vi "logo.vi"() -> ()   [LabVIEW 2015]
panel:
  in  "Run!":bool
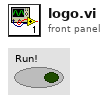
[diagram p1: front panel]
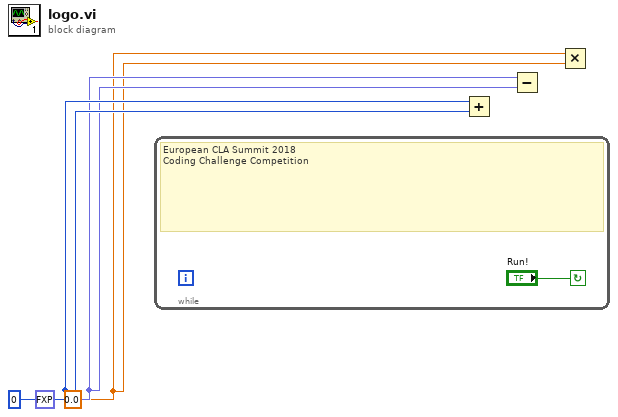
[diagram p0: block diagram]
diagram:
  w1 = 0.0 ("y")
  w2 = fxp<+,1,1> 0.0 ("y")
  w3 = 0
  n1 = while {
    stop <- "Run!" continue-if-true
    # "European CLA Summit 2018\nCoding Challenge Competition"
  }
  n2 = Add(x=w3, y=w3) -> ()  [unwired: 1 out]
  n3 = Subtract(x=w2, y=w2) -> ()  [unwired: 1 out]
  n4 = Multiply(x=w1, y=w1) -> ()  [unwired: 1 out]
